vi "RFSA Frequency Sweep in SW.vi"() -> ()   [LabVIEW 2017]
doc: "Demonstrates how to acquire a spectrum using the RF vector signal analyzer. This example shows how to configure NI-RFSA for spectrum acquisition, how to set the resolution bandwidth and reference level, and how to read power spectra while changing the center frequency in each iteration of the sweep while keeping the span constant. The spectrum is displayed on the graph. <B>Note</B> This example illustrates how to perform multiple spectrum acquisitions with different center frequency values. If you need to acquire a spectrum with a span wider than the instantaneous bandwidth of the device, use the Getting Started Spectrum example."
uses:
  <vilib>/Utility/error.llb/DialogType.ctl
  <vilib>/Analysis/1siggen.llb/Ramp Pattern by Delta.vi
  <instrlib>/niRFSA/niRFSA.llb/niRFSA Read Power Spectrum (DBL).vi
  <vilib>/Analysis/NI_AALBase.lvlib
panel:
  out "size(s)":i32
  in  "delta":dbl format="%#_6p"
  out "Ramp Pattern":dbl[](array[numeric]) format="%#_6p"
  in  "stop":bool
  in  "Resource Name":refnum<k15>="RFSA"
  in  "Start Center Frequency (Hz)":dbl=990000000.0 format="%#.3p"
  in  "Stop Center Frequency (Hz)":dbl=1010000000.0 format="%#.3p"
  in  "Span (Hz)":dbl=20000000.0 format="%#.3p"
  out "Current Center Frequency":dbl=1010000000.0 format="%#.3p"
  out "Power Spectrum":cluster{"f0":dbl, "df":dbl, "data":dbl[]}(graph)={"f0"=1000024038.4615384, "df"=40064.10256410256, "data"=[]}
  in  "Resolution Bandwidth (Hz)":dbl=100000.0 format="%#.3p"
  in  "Reference Level (dBm)":dbl format="%.2f"
  # "Overview: Demonstrates how to acquire a spectrum using the RF vector signal analyzer. \nRequirements: NI-RFSA\nInstructions:\n1. Change the Resource Name to your device.\n2. Run the VI.\n3. Click Stop to stop the VI."
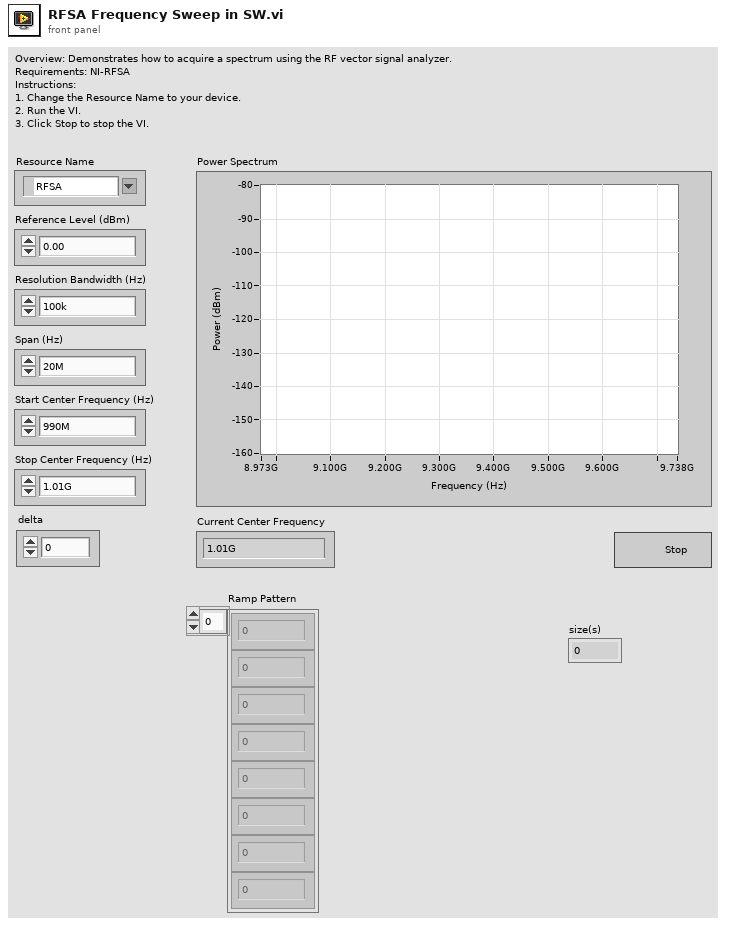
[diagram p1: front panel]
types:
  T1 = typedef "DialogType.ctl" = u16
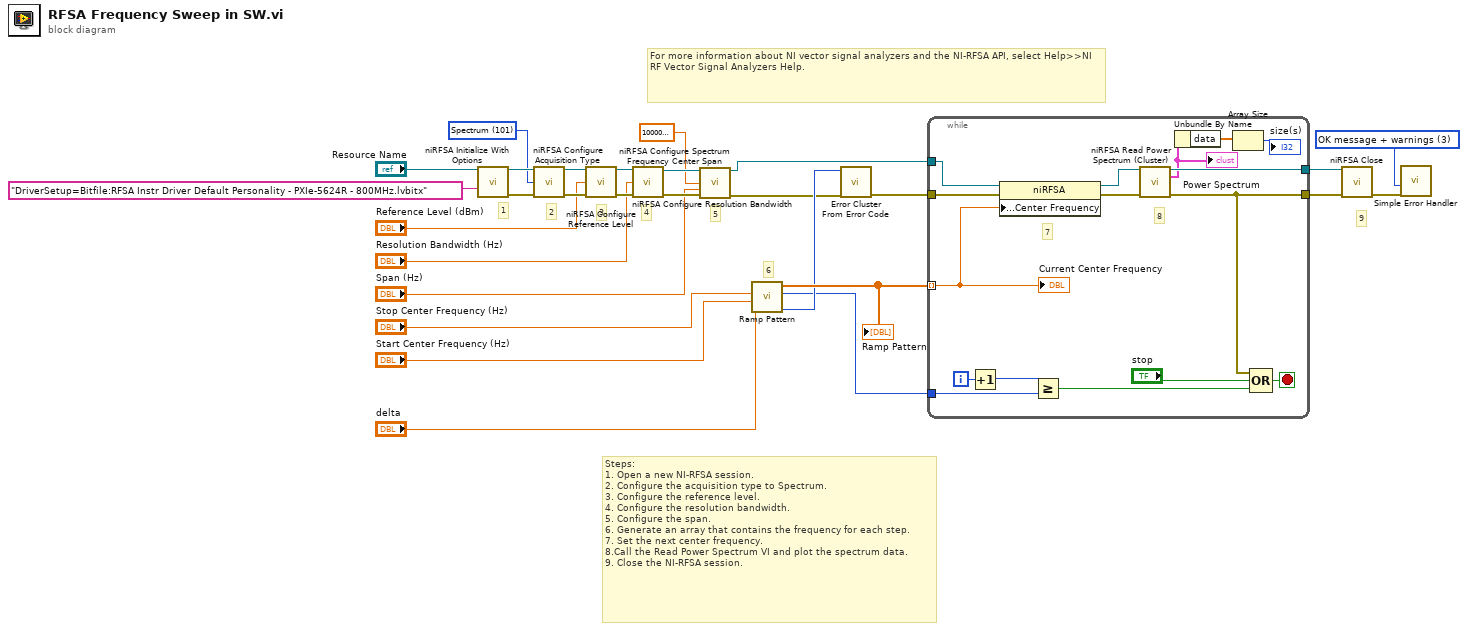
[diagram p0: block diagram]
diagram:
  w14 = T1 3 items=["no dialog", "OK message", "continue or stop message", "OK message + warnings", "continue/stop + warnings"] ("type of dialog (OK msg:1)")
  w16 = 101 items=["IQ"=100, "Spectrum"=101] ("Acquisition:Acquisition Type")
  # "For more information about NI vector signal analyzers and the NI-RFSA API, select Help>>NI  RF Vector Signal Analyzers Help."
  # "9"
  # "6"
  # "5"
  # "4"
  # "3"
  # "2"
  # "1"
  # "Steps:\n1. Open a new NI-RFSA session.\n2. Configure the acquisition type to Spectrum.\n3. Configure the reference level.\n4. Configure the resolution bandwidth.\n5. Configure the span.\n6. Generate an array that contains the frequency for each step.\n7. Set the next center frequency.\n8.Call the Read Power Spectrum VI and plot the spectrum data.\n9. Close the NI-RFSA session."
  n1 = call <instrlib>:"niRFSA Initialize With Options.vi"("resource name"="Resource Name", "option string"="DriverSetup=Bitfile:RFSA Instr Driver Default Personality - PXIe-5624R - 800MHz.lvbitx") -> ("instrument handle out"=w26:refnum<k15>, "error out"=w25:errorcluster)  [unwired: 12 in]
  n2 = call <instrlib>:"niRFSA Configure Acquisition Type.vi"("instrument handle"=w26, "acquisition type"=w16, "error in"=w25) -> ("instrument handle out"=w23:refnum<k15>, "error out"=w24:errorcluster)  [unwired: 11 in]
  n3 = call <instrlib>:"niRFSA Configure Reference Level.vi"("instrument handle"=w23, "reference level (dBm)"="Reference Level (dBm)", "error in"=w24) -> ("instrument handle out"=w20:refnum<k15>, "error out"=w19:errorcluster)  [unwired: 11 in]
  n4 = call <instrlib>:"niRFSA Configure Resolution Bandwidth.vi"("instrument handle"=w20, "resolution bandwidth (Hz)"="Resolution Bandwidth (Hz)", "error in"=w19) -> ("instrument handle out"=w21:refnum<k15>, "error out"=w18:errorcluster)  [unwired: 11 in]
  n5 = call <instrlib>:"niRFSA Configure Spectrum Frequency Center Span.vi"("instrument handle"=w21, "frequency"=100000000.0, "span"="Span (Hz)", "error in"=w18) -> ("instrument handle out"=w17:refnum<k15>, "error out"=w7:errorcluster)  [unwired: 10 in]
  n6 = call-poly <vilib>:"Ramp Pattern.vi"("start"="Start Center Frequency (Hz)", "end"="Stop Center Frequency (Hz)", "delta"="delta") -> ("error"=w8:i32, "samples"=w1:i32, "Ramp Pattern"=w28:dbl[])  [unwired: 6 in]
  "Ramp Pattern" <- w28
  n7 = call <vilib>:"Error Cluster From Error Code.vi"("error in (no error)"=w7, "error code (0)"=w8) -> ("error out"=w6:errorcluster)  [unwired: 7 in]
  n8 = while {
    tunnel: w28 -> [w41] mode=indexing
    tunnel: w1 -> [w44]
    tunnel: w17 -> [w40]
    tunnel: [w37] -> w27
    tunnel: w6 -> [w33]
    tunnel: [w32] -> w5
    i -> [w43]
    stop <- w36 stop-if-true
    # "8"
    # "7"
    n9 = Increment(x=w43) -> (x+1=w42:i32)
    n10 = property class="niRFSA"(reference=w40, error in=w33, "Acquisition:Spectrum:Center Frequency"=w41) -> (reference out=w39:refnum<k15>, error out=w38:errorcluster)
    n11 = Greater Or Equal?(x=w42, y=w44) -> (x >= y?=w35:bool)
    n12 = call-poly <instrlib>:"niRFSA Read Power Spectrum (Cluster).vi"("instrument handle"=w39, "error in"=w38) -> ("instrument handle out"=w37:refnum<k15>, "power spectrum"=w31:cluster{"f0":dbl, "df":dbl, "data":dbl[]}, "error out"=w32:errorcluster)  [unwired: 11 in]
    "Power Spectrum" <- w31
    n13 = Unbundle By Name(w31) -> ("data"=w30:dbl[])
    n14 = Array Size(array=w30) -> (size(s)=→"size(s)":i32)
    n15 = Compound Arithmetic op=OR(w32, "stop", w35) -> (w36:bool)
    "Current Center Frequency" <- w41
  }
  n16 = call <instrlib>:"niRFSA Close.vi"("instrument handle"=w27, "error in"=w5) -> ("error out"=w22:errorcluster)  [unwired: 13 in]
  n17 = call <vilib>:"Simple Error Handler.vi"("type of dialog (OK msg:1)"=w14, "error in (no error)"=w22) -> ()  [unwired: 3 in, 5 out]
